vi "LoadEyeArray.vi"(0 "directory path of data and header file":path, 1 "Split files?":bool, 3 "Type of Read":T2(ring)=enum."Save IQSum", 5 "String":string="*_HeaderInfoRcv.txt", 7 "Only Buff 3?":bool, 12 "Only Real of Sum?":bool, 13 "Cut off":i32=50000) -> (4 "RcvBuff 3":cdb[][][](array[numeric]), 6 "output array":i32[][][](array[numeric]), 8 "Header Out":T1={"header info"={"Header"="", "Head length"=0}, "A/D info"={"# rf points per line"=0, "# lines per scan"=0, "sample rate MHz"=0, "# A/D bits"=0, "# bytes per A/D"=0, "TGC Flag"=0, "A/D Type"=""}, "Tranducer Info"={"bandwidth"=0.0, "center freq"=0.0, "start freq"=0.0, "ID"=0}, "Scan Info"={"delay"=0.0, "pivot distance"=0.0, "sector scan angle"=0.0, "operator"="", "Scan Mode"="", "location"=""}, "Time/Date Info"={"date"="", "time"=""}, "RF Info"={"RF file name"="", "RF file att"="", "RF cal file name"="", "RF cal file att"=""}, "Patient Info"={"ID"="", "extended ID"="", "age"=0, "sex"="", "previously\nscanned"="", "PSA"=0.0, "LOS"=1, "Ethnicty 2"=3, "Race"=3}, "Tissue Type"={"organ"=0, "disease type"=0, "disease location"=0, "IQ_pts"=0, "RcvBuffer"=0, "RcvFrame"=0, "IQBuff"=0, "IQFrame"=0, "IQPage"=0}, "Votage scaling"={"Digitizer (dB)"=0.0, "Gain (dB)"=0.0, "Atten (dB)"=0.0}, "Comment"="", "Misc Info"={"avg num"=0, "c speed"=0, "Div By or SF zones"=0, "XMIT CHS"=0, "RCV CHS"=0, "Xmit angle"=0.0}, "Therapy Parameters"={"Theraputic Freq (MHz)"=0.0, "Time on (s)"=0.0, "Therapy amplitude (mV)"=0.0, "Lines Before"=0, "Lines After"=0}, "Scan Settings"={"Energy (uJ or V)"=0, "Damp (Ohm) or Fc"=0, "HP Filt (KHz)"=0, "LP Filt (MHz)"=0, "Gain (db)"=0, "prf (kHz)"=0.0, "Distance between\nscan lines (um)"=0, "Distance between\nscan planes (um)"=0, "Scan line gap (um)"=0.0, "Scan plane gap (um)"=0.0}, "Compression Parameters"={"F1 (MHz)"=0.0, "F2 (MHz)"=0.0, "% taper"=0.0, "duration"=0.0}, "Patient Info Xtra"={"First Name"="", "Last Name"="", "Notes"=""}, "ROI Box"=[0, 0, 0, 0]} {"Compression Parameters"."% taper" min=50 max=1000 format="%.2f"; "Compression Parameters"."F2 (MHz)" format="%.3f"; "Compression Parameters"."F1 (MHz)" format="%.3f"; "Scan Settings"."prf (kHz)" format="%.2f"; "Therapy Parameters"."Therapy amplitude (mV)" min=50 max=1000 format="%.2f"; "Therapy Parameters"."Time on (s)" format="%.3f"; "Therapy Parameters"."Theraputic Freq (MHz)" format="%.3f"; "Patient Info"."Race" items=["Am Ind or Alaska", "Asian", "Hawaiian, Pac Isl", "Black or Afr Amer", "White", "more than one race", "unknown"]; "Patient Info"."Ethnicty 2" items=["Hispanic", "Non-Hispanic", "unknown"]; "Patient Info"."LOS" items=["1", "2", "3", "4", "5"]; "Patient Info"."PSA" format="%.1f"; "Scan Info"."delay" format="%.2f"; "Scan Info"."pivot distance" format="%.2f"; "Scan Info"."sector scan angle" format="%.2f"; "Tranducer Info"."bandwidth" format="%.2f"; "Tranducer Info"."center freq" format="%.2f"; "Tranducer Info"."start freq" format="%.2f"}, 10 "time diff (25 us time steps)":sgl[](graph), 15 "time stamp":sgl[](graph))   [LabVIEW 2022 SP3]
uses:
  ViewData/-ReadEye/Header.ctl
  <vilib>/Utility/file.llb/Read Delimited Spreadsheet (string).vi
  <vilib>/Utility/file.llb/Read Delimited Spreadsheet (DBL).vi
  <userlib>/_OpenG.lib/array/array.llb/Sort 2D Array (DBL)__ogtk.vi
panel:
  in  "#Sets":i32=1 min=1 max=100 step=1
  in  "Extra Char":string
  out "Raw data":dbl[][](graph)
  out "Current File":string
  in  "IQ source":enum32{"GPU", "Verasonics", "None"}(radio)
  out "Current File Ct":i32
  out "Header Size":i32[](array[numeric])
  out "Header clolumn names":string[](array[string])
  in  "Header as cluster":T3
  out "Header Values sorted":dbl[][](array[numeric])
  # "Naming must match up\nDo not change order in Matlab save !!!!!!!!!!!!!!!!!!!!!!!!!!!!!!"
  # "For LoopCT can add in _0n for the raw case"
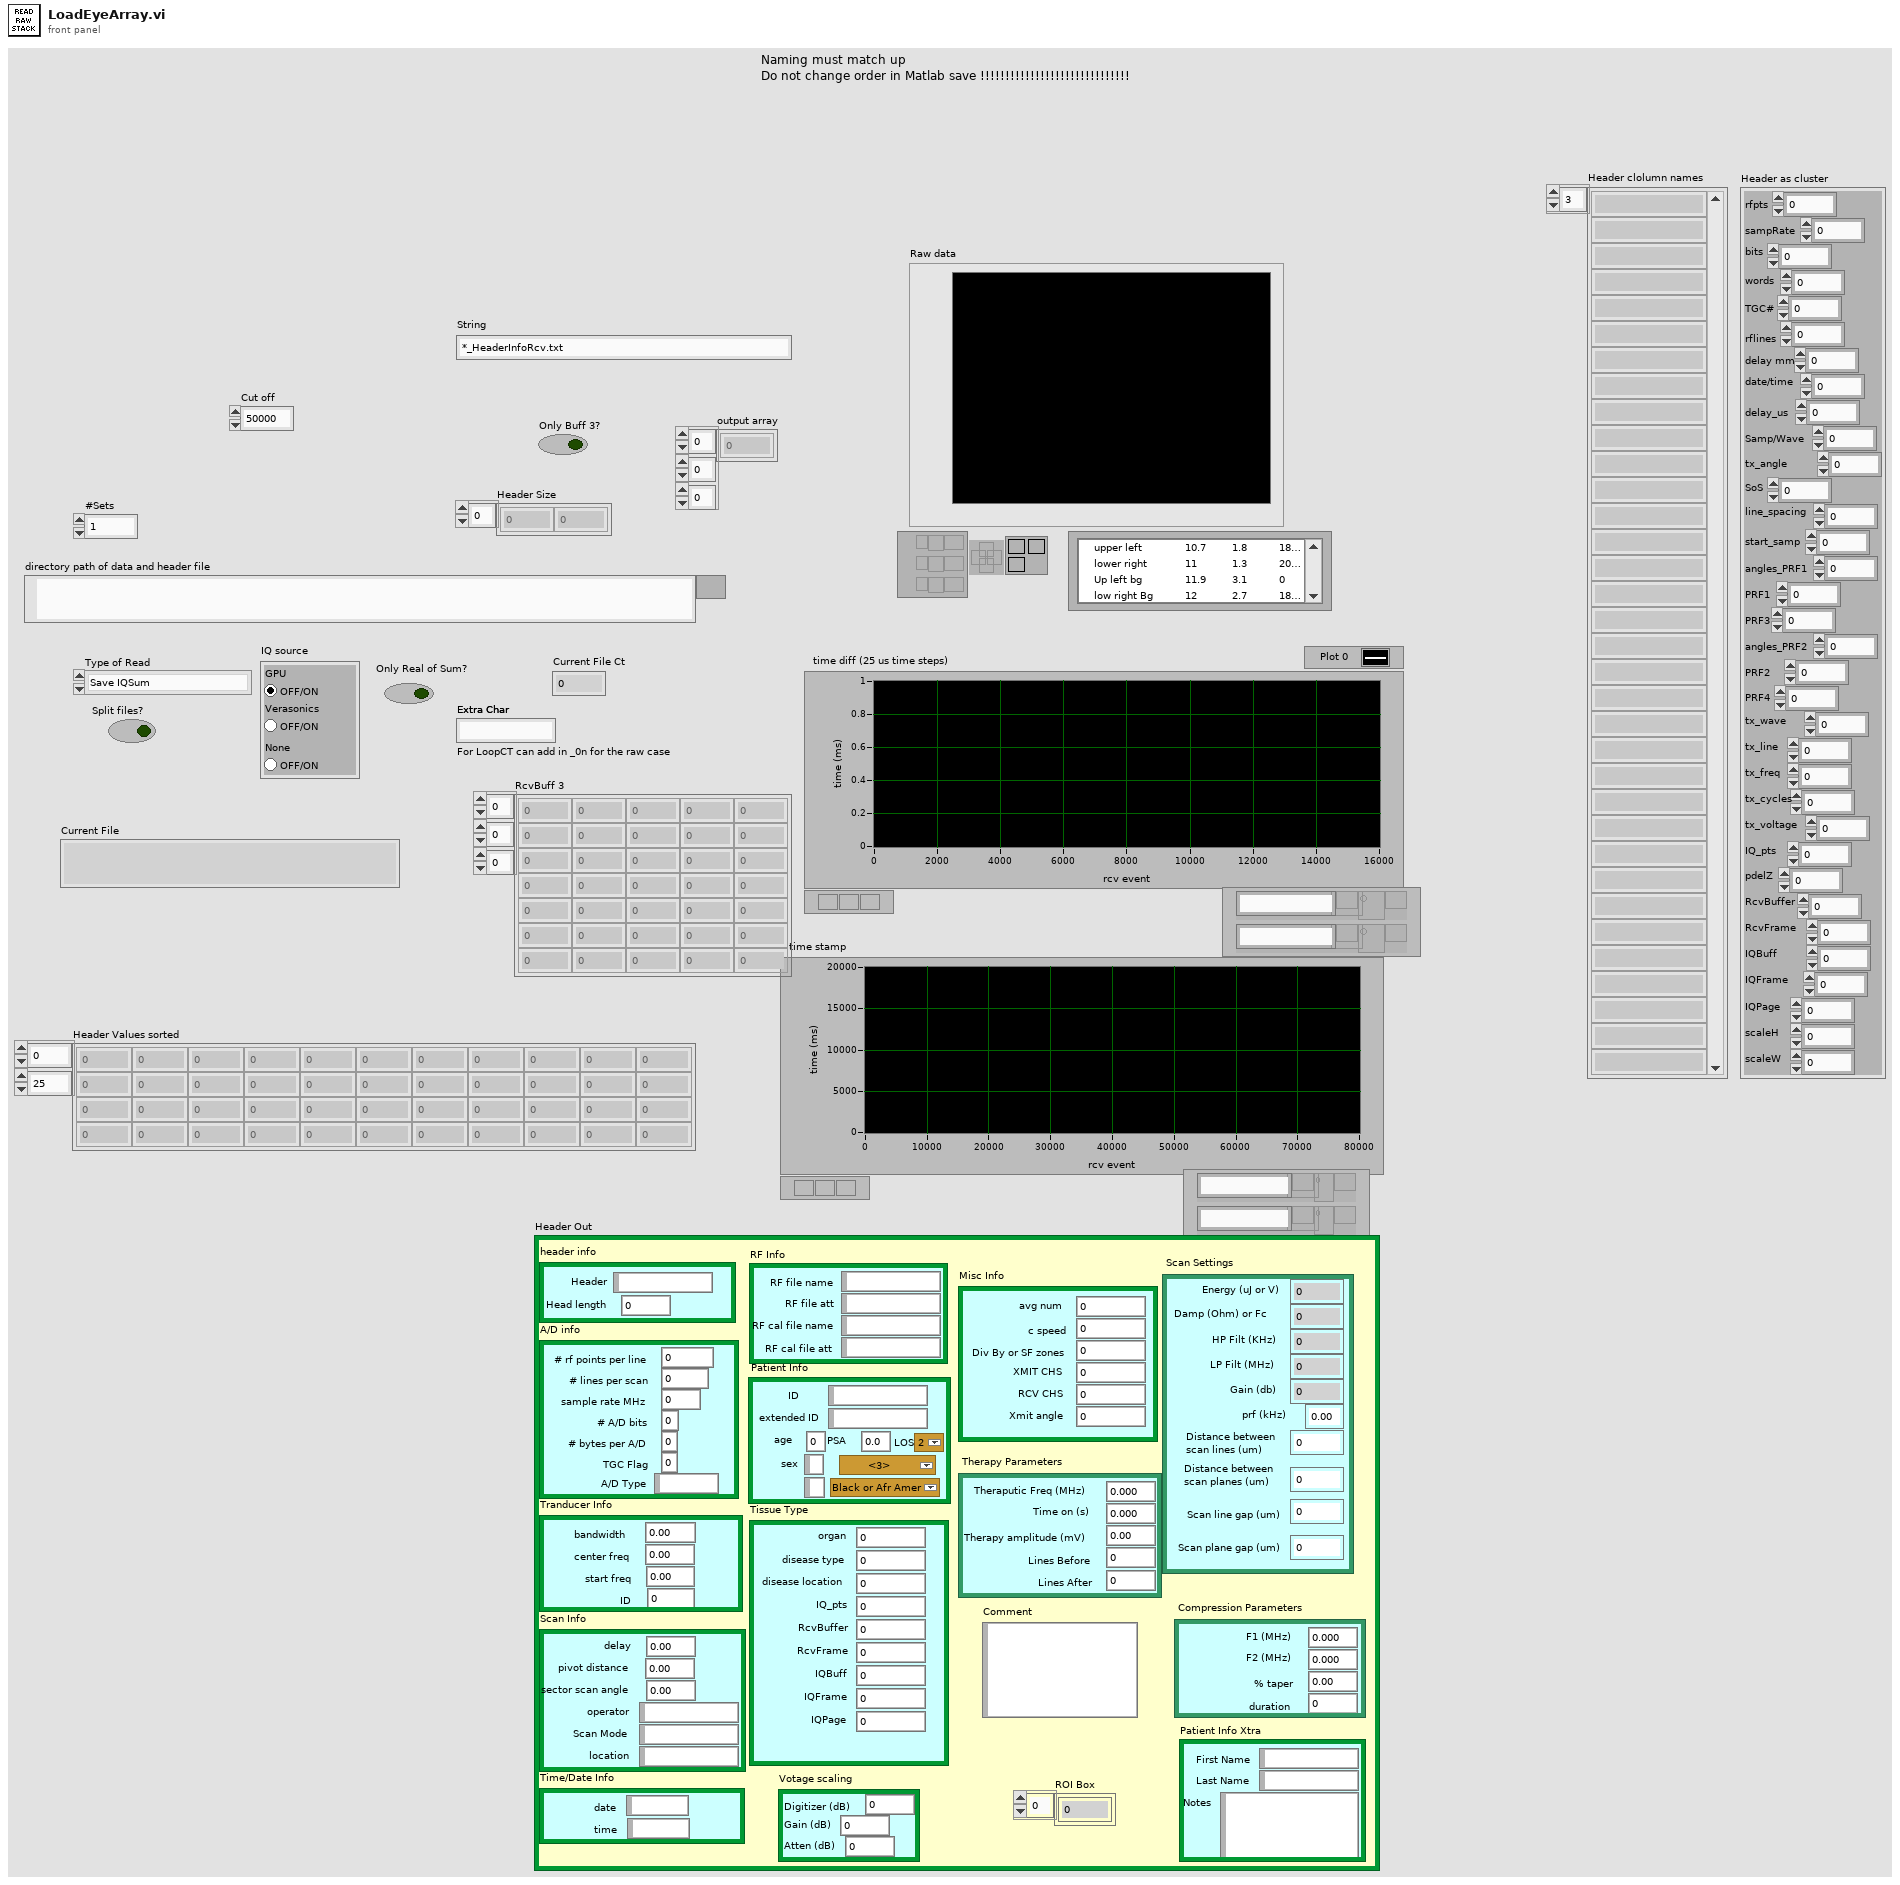
[diagram p1: front panel]
types:
  T1 = typedef "Header.ctl" = cluster{"header info":cluster{"Header":string, "Head length":i16}, "A/D info":cluster{"# rf points per line":u16, "# lines per scan":u16, "sample rate MHz":u16, "# A/D bits":i16, "# bytes per A/D":u16, "TGC Flag":u16, "A/D Type":string}, "Tranducer Info":cluster{"bandwidth":sgl, "center freq":sgl, "start freq":sgl, "ID":i32}, "Scan Info":cluster{"delay":sgl, "pivot distance":sgl, "sector scan angle":sgl, "operator":string, "Scan Mode":string, "location":string}, "Time/Date Info":cluster{"date":string, "time":string}, "RF Info":cluster{"RF file name":string, "RF file att":string, "RF cal file name":string, "RF cal file att":string}, "Patient Info":cluster{"ID":string, "extended ID":string, "age":u16, "sex":string, "previously\nscanned":string, "PSA":sgl, "LOS":u8, "Ethnicty 2":u8, "Race":u8}, "Tissue Type":cluster{"organ":i16, "disease type":i16, "disease location":i16, "IQ_pts":u16, "RcvBuffer":u8, "RcvFrame":u16, "IQBuff":u8, "IQFrame":u16, "IQPage":u8}, "Votage scaling":cluster{"Digitizer (dB)":sgl, "Gain (dB)":sgl, "Atten (dB)":sgl}, "Comment":string, "Misc Info":cluster{"avg num":u16, "c speed":i16, "Div By or SF zones":i16, "XMIT CHS":u8, "RCV CHS":u8, "Xmit angle":sgl}, "Therapy Parameters":cluster{"Theraputic Freq (MHz)":sgl, "Time on (s)":sgl, "Therapy amplitude (mV)":sgl, "Lines Before":u16, "Lines After":u16}, "Scan Settings":cluster{"Energy (uJ or V)":u8, "Damp (Ohm) or Fc":u8, "HP Filt (KHz)":u8, "LP Filt (MHz)":u8, "Gain (db)":u8, "prf (kHz)":sgl, "Distance between\nscan lines (um)":u16, "Distance between\nscan planes (um)":u16, "Scan line gap (um)":sgl, "Scan plane gap (um)":sgl}, "Compression Parameters":cluster{"F1 (MHz)":sgl, "F2 (MHz)":sgl, "% taper":sgl, "duration":sgl}, "Patient Info Xtra":cluster{"First Name":string, "Last Name":string, "Notes":string}, "ROI Box":u16[]}
  T2 = enum16{"None", "Raw RF + time stamp", "Save IQAll", "Save IQSum", "Save IQSumReal", "Save Img", "Time Stamps", "unused"}
  T3 = cluster{"rfpts":dbl, "sampRate":dbl, "bits":dbl, "words":dbl, "TGC#":dbl, "rflines":dbl, "delay mm":dbl, "date/time":dbl, "delay_us":dbl, "Samp/Wave":dbl, "tx_angle":dbl, "SoS":dbl, "line_spacing":dbl, "start_samp":dbl, "angles_PRF1":dbl, "PRF1":dbl, "PRF3":dbl, "angles_PRF2":dbl, "PRF2":dbl, "PRF4":dbl, "tx_wave":dbl, "tx_line":dbl, "tx_freq":dbl, "tx_cycles":dbl, "tx_voltage":dbl, "IQ_pts":dbl, "pdelZ":dbl, "RcvBuffer":dbl, "RcvFrame":dbl, "IQBuff":dbl, "IQFrame":dbl, "IQPage":dbl, "scaleH":dbl, "scaleW":dbl}
  T4 = enum16{"big-endian, network order", "native, host order", "little-endian"}
  T5 = cluster{"Sorted Array out[0]":dbl, "Sorted Array out[1]":dbl, "Sorted Array out[2]":dbl, "Sorted Array out[3]":dbl, "Sorted Array out[4]":dbl, "Sorted Array out[5]":dbl, "Sorted Array out[6]":dbl, "Sorted Array out[7]":dbl, "Sorted Array out[8]":dbl, "Sorted Array out[9]":dbl, "Sorted Array out[10]":dbl, "Sorted Array out[11]":dbl, "Sorted Array out[12]":dbl, "Sorted Array out[13]":dbl, "Sorted Array out[14]":dbl, "Sorted Array out[15]":dbl, "Sorted Array out[16]":dbl, "Sorted Array out[17]":dbl, "Sorted Array out[18]":dbl, "Sorted Array out[19]":dbl, "Sorted Array out[20]":dbl, "Sorted Array out[21]":dbl, "Sorted Array out[22]":dbl, "Sorted Array out[23]":dbl, "Sorted Array out[24]":dbl, "Sorted Array out[25]":dbl, "Sorted Array out[26]":dbl, "Sorted Array out[27]":dbl, "Sorted Array out[28]":dbl, "Sorted Array out[29]":dbl, "Sorted Array out[30]":dbl, "Sorted Array out[31]":dbl, "Sorted Array out[32]":dbl, "Sorted Array out[33]":dbl, "Sorted Array out[34]":dbl}
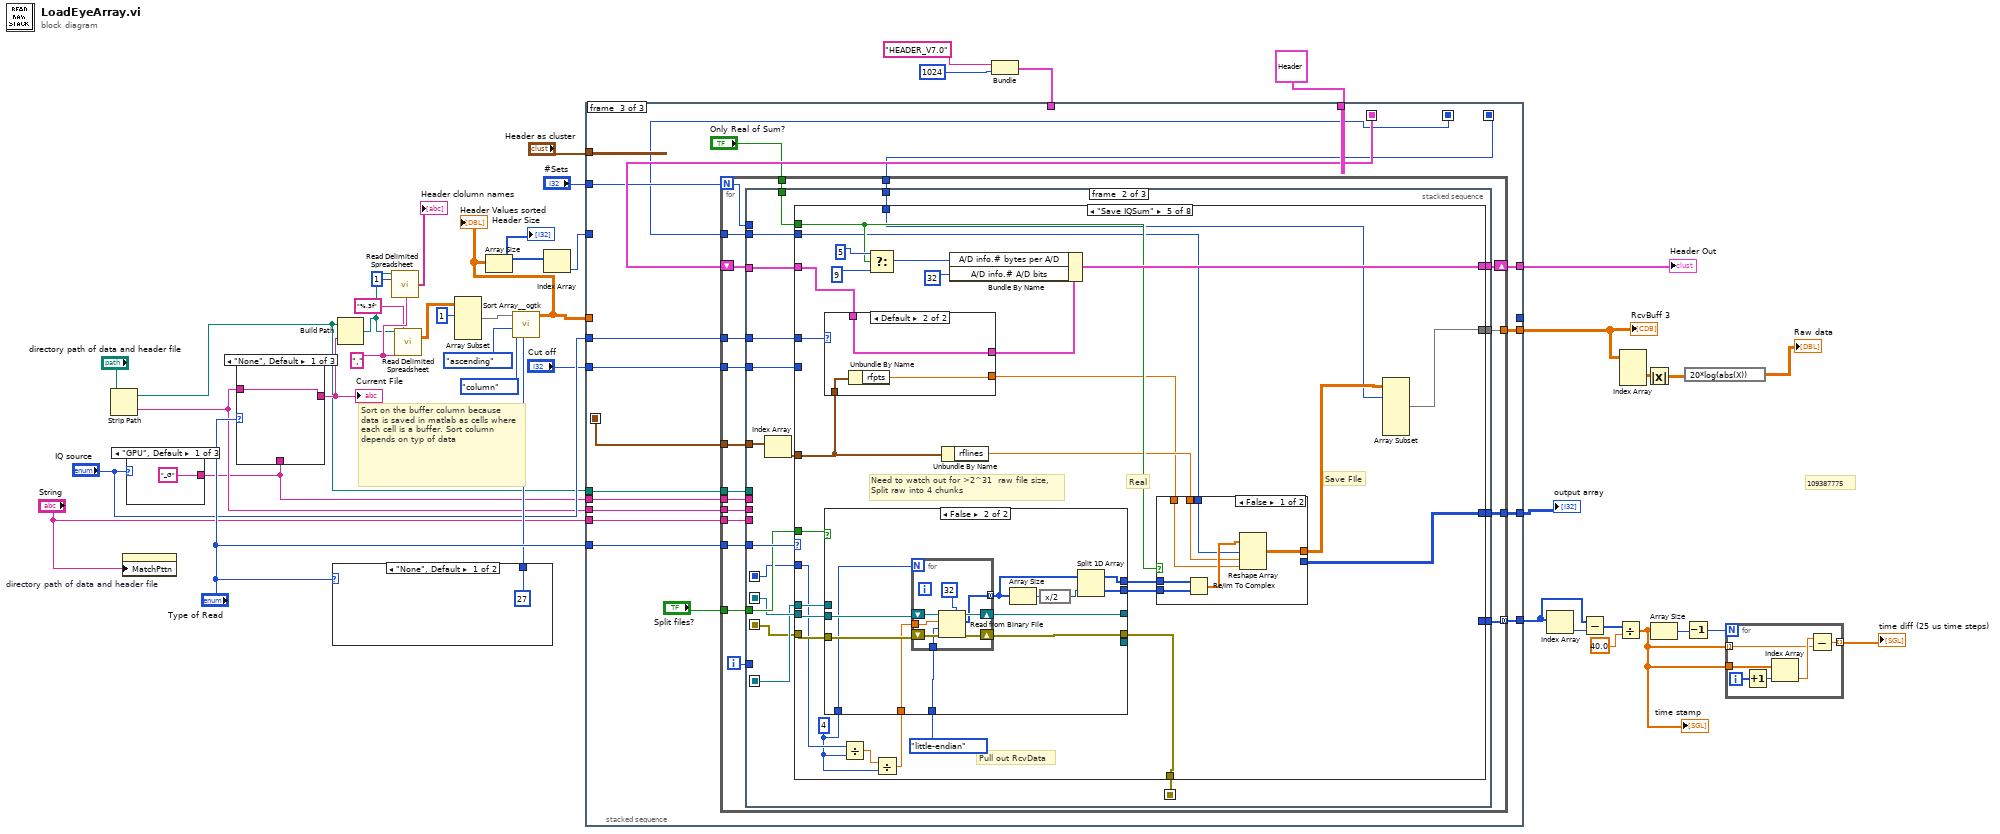
[diagram p0: block diagram]
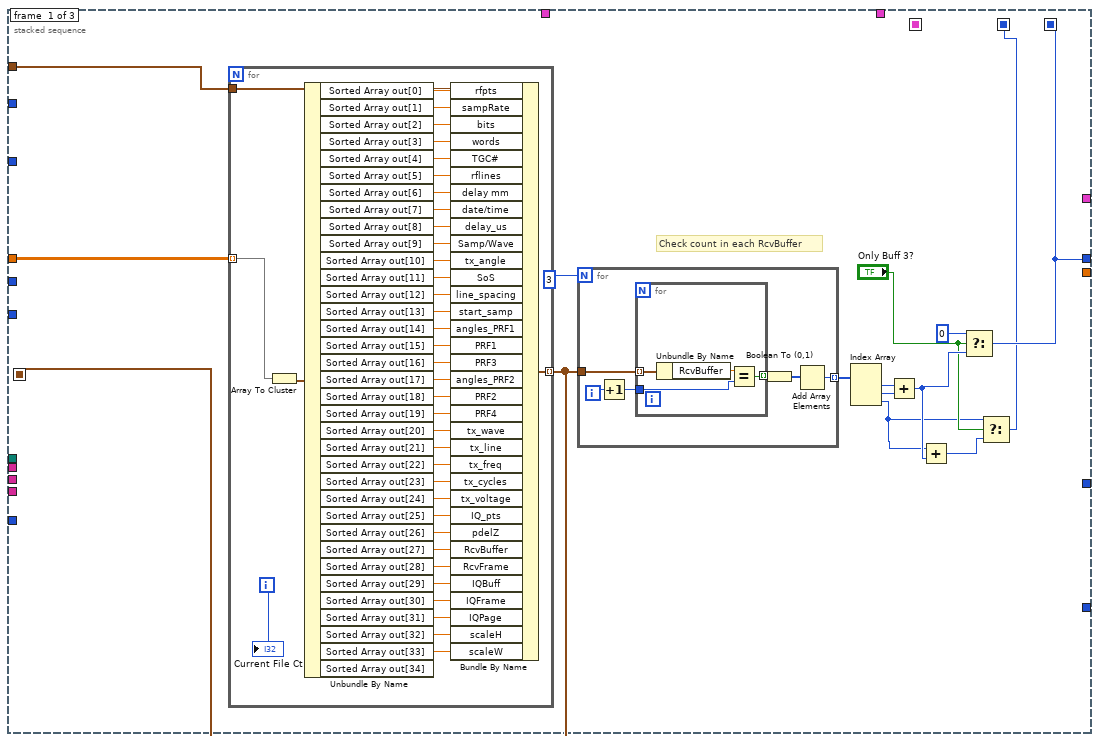
[diagram p2: hidden frame]
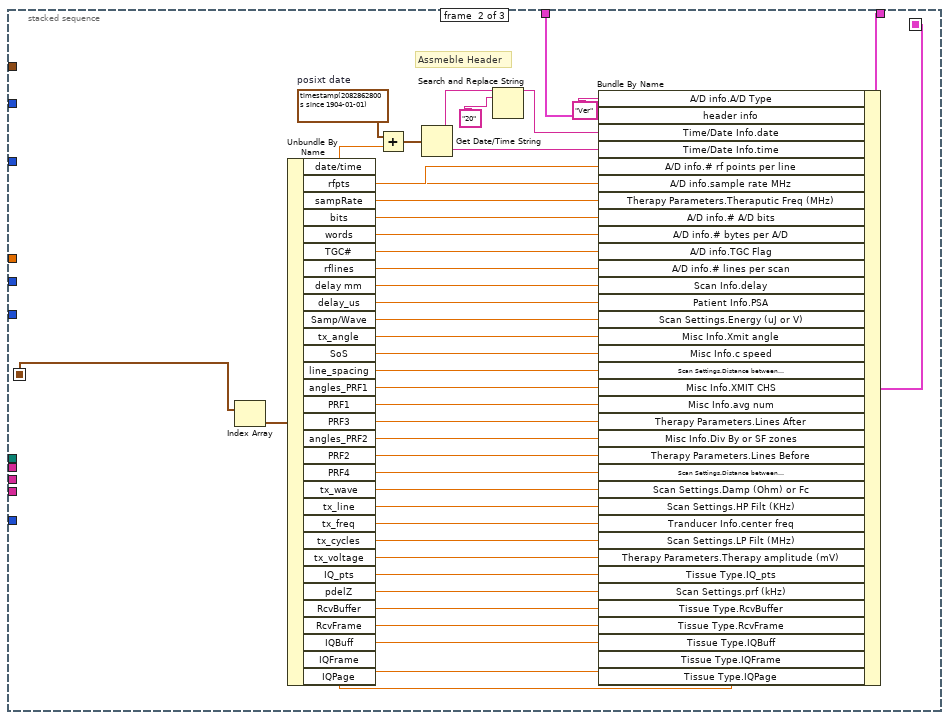
[diagram p3: hidden frame]
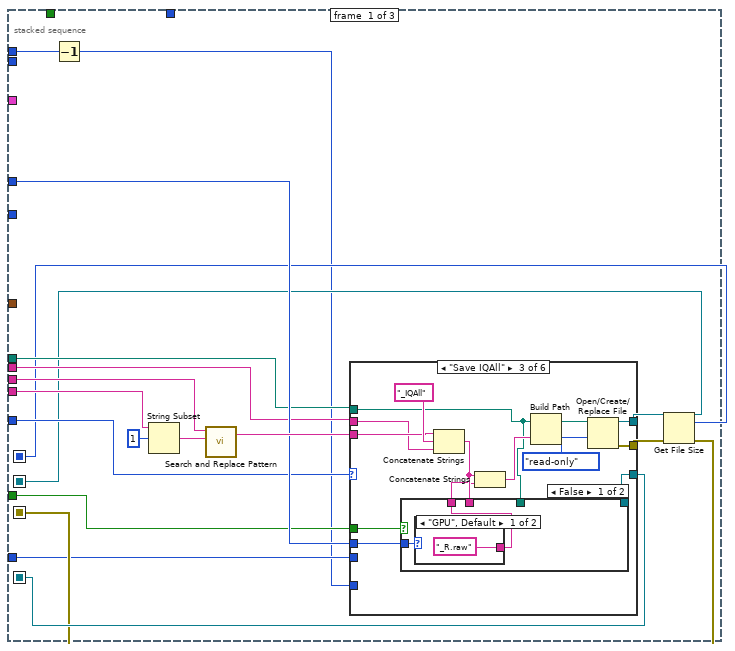
[diagram p4: hidden frame]
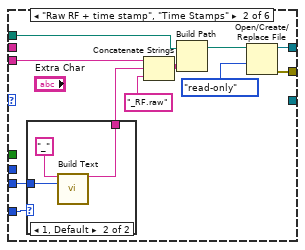
[diagram p6: hidden frame]
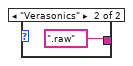
[diagram p8: hidden frame]
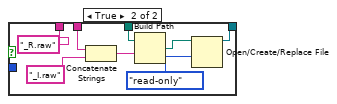
[diagram p9: hidden frame]
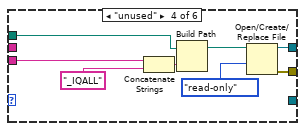
[diagram p10: hidden frame]
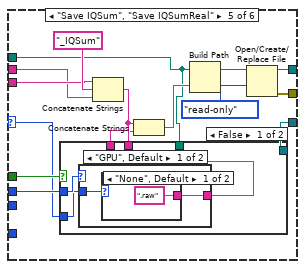
[diagram p11: hidden frame]
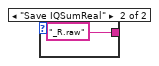
[diagram p12: hidden frame]
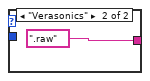
[diagram p13: hidden frame]
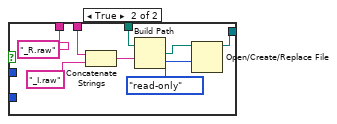
[diagram p14: hidden frame]
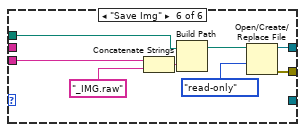
[diagram p15: hidden frame]
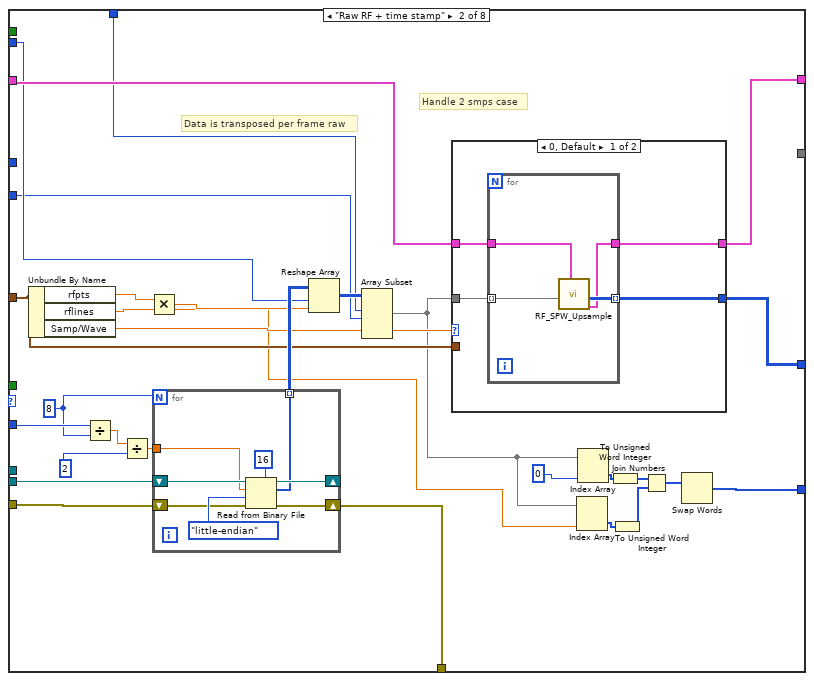
[diagram p17: hidden frame]
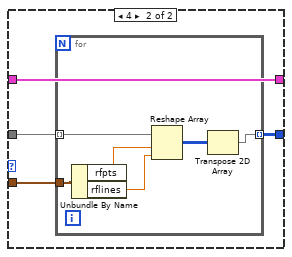
[diagram p18: hidden frame]
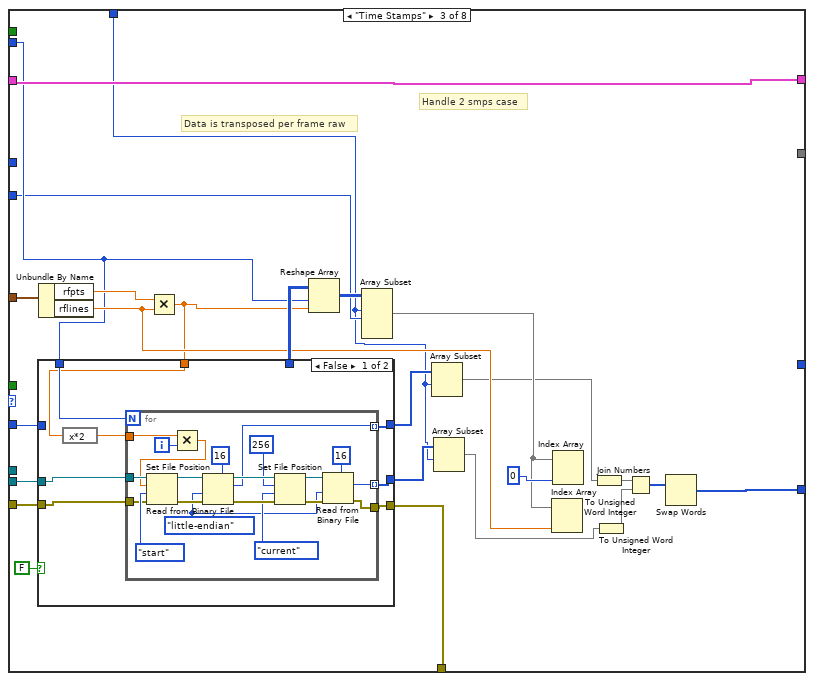
[diagram p19: hidden frame]
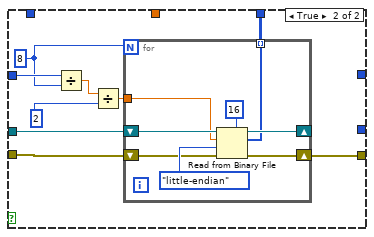
[diagram p20: hidden frame]
diagram:
  w34 = "," ("delimiter (\\t)")
  # "109387775"
  # "Sort on the buffer column because data is saved in matlab as cells where each cell is a buffer. Sort column depends on typ of data"
  n1 = Strip Path(path="directory path of data and header file") -> (stripped path=w11:path, name=w13:string)
  n2 = property on="directory path of data and header file" class="Path"("MatchPttn"="String") -> ()  [unwired: 2 in, 2 out]
  n3 = case shown="\"GPU\", Default" "IQ source" {
    tunnel: ["_G" ("replace string (\"\")") "_V" ("replace string (\"\")") _] -> w12
    frame "GPU", Default {
    }
    frame "Verasonics" {
    }
    frame "None" {
    }
  }
  n4 = case shown="\"None\", Default" "Type of Read" {
    tunnel: w13 -> [w46 w51 w57]
    tunnel: [w46 w50 w56] -> w31
    tunnel: w12 -> [_ w47 w53]
    frame "None", Default {
    }
    frame "Save IQSum".."Save Img" {
      n5 = Concatenate Strings("IQSum" ("replace string (\"\")"), w47) -> (w48:string)
      n6 = Search and Replace String(input string=w51, search string="Rcv", replace string=w48) -> (result string=w50:string)  [unwired: 5 in, 3 out]
    }
    frame "Save IQAll" {
      n7 = Concatenate Strings("IQAll" ("replace string (\"\")"), w53) -> (w54:string)
      n8 = Search and Replace String(input string=w57, search string="Rcv", replace string=w54) -> (result string=w56:string)  [unwired: 5 in, 3 out]
    }
  }
  "Current File" <- w31
  n9 = case shown="\"None\", Default" "Type of Read" {
    tunnel: [u32 27 ("Column/Row to Sort By") u32 29 ("Column/Row to Sort By")] -> w26
    frame "None", Default {
    }
    frame "Save IQSum".."Save Img" {
    }
  }
  n10 = Build Path(base path=w11, name or relative path=w31) -> (appended path=w23:path)
  n11 = call-poly <vilib>:"Read Delimited Spreadsheet.vi"("file path (dialog if empty)"=w23, "number of rows (all:-1)"=1, "delimiter (\\t)"=w34) -> ("first row"=→"Header clolumn names":string[])  [unwired: 7 in, 5 out]
  n12 = call-poly <vilib>:"Read Delimited Spreadsheet.vi"("file path (dialog if empty)"=w23, "format (%.3f)"="%.3f", "delimiter (\\t)"=w34) -> ("all rows"=w37:dbl[][])  [unwired: 7 in, 5 out]
  n13 = Array Subset(array=w37, index (row)=1 ("index")) -> (w28:dbl[][])  [unwired: 3 in]
  n14 = call-poly <userlib>:"Sort Array__ogtk.vi"("Column/Row to Sort By"=w26, "Sort By in"=enum16{"row", "column"}."column", "Order"=enum16{"ascending", "descending"}."ascending", "Array in"=w28) -> ("Sorted Array out"=w27:dbl[][])  [unwired: 4 in, 3 out]
  "Header Values sorted" <- w27
  n15 = Array Size(array=w27) -> (size(s)=w22:i32[])
  "Header Size" <- w22
  n16 = Index Array(array=w22) -> (element=w9:i32)  [unwired: 1 in]
  n17 = Bundle("HEADER_V7.0", 1024) -> (w40:cluster{string, i32})  [unwired: 1 in]
  n18 = stacked-sequence {
    seq-local: [_ w135 _] -> [_ _ w184]
    seq-local: [w71 _ _] -> [_ w125 w177]
    seq-local: [w65 _ _] -> [_ _ w176]
    seq-local: [w61 _ _] -> [_ _ w167]
    tunnel: T1 {"header info"={"Header"="", "Head length"=0}, "A/D info"={"# rf points per line"=0, "# lines per scan"=0, "sample rate MHz"=0, "# A/D bits"=0, "# bytes per A/D"=0, "TGC Flag"=0, "A/D Type"=""}, "Tranducer Info"={"bandwidth"=0.0, "center freq"=0.0, "start freq"=0.0, "ID"=0}, "Scan Info"={"delay"=0.0, "pivot distance"=0.0, "sector scan angle"=0.0, "operator"="", "Scan Mode"="", "location"=""}, "Time/Date Info"={"date"="", "time"=""}, "RF Info"={"RF file name"="", "RF file att"="", "RF cal file name"="", "RF cal file att"=""}, "Patient Info"={"ID"="", "extended ID"="", "age"=0, "sex"="", "previously\nscanned"="", "PSA"=0.0, "LOS"=1, "Ethnicty 2"=3, "Race"=3}, "Tissue Type"={"organ"=0, "disease type"=0, "disease location"=0, "IQ_pts"=0, "RcvBuffer"=0, "RcvFrame"=0, "IQBuff"=0, "IQFrame"=0, "IQPage"=0}, "Votage scaling"={"Digitizer (dB)"=0.0, "Gain (dB)"=0.0, "Atten (dB)"=0.0}, "Comment"="", "Misc Info"={"avg num"=0, "c speed"=0, "Div By or SF zones"=0, "XMIT CHS"=0, "RCV CHS"=0, "Xmit angle"=0.0}, "Therapy Parameters"={"Theraputic Freq (MHz)"=0.0, "Time on (s)"=0.0, "Therapy amplitude (mV)"=0.0, "Lines Before"=0, "Lines After"=0}, "Scan Settings"={"Energy (uJ or V)"=0, "Damp (Ohm) or Fc"=0, "HP Filt (KHz)"=0, "LP Filt (MHz)"=0, "Gain (db)"=0, "prf (kHz)"=0.0, "Distance between\nscan lines (um)"=0, "Distance between\nscan planes (um)"=0, "Scan line gap (um)"=0.0, "Scan plane gap (um)"=0.0}, "Compression Parameters"={"F1 (MHz)"=0.0, "F2 (MHz)"=0.0, "% taper"=0.0, "duration"=0.0}, "Patient Info Xtra"={"First Name"="", "Last Name"="", "Notes"=""}, "ROI Box"=[0, 0, 0, 0]} ("Header In") -> [_ w166 _]
    tunnel: w40 -> [_ w140 _]
    tunnel: "Type of Read" -> [_ _ w183]
    tunnel: w27 -> [w74 _ _]
    tunnel: "Header as cluster" -> [w73 _ _]
    tunnel: "IQ source" -> [_ _ w182]
    tunnel: [_ _ w180] -> w38
    tunnel: w9 -> [_ _ _]
    tunnel: [_ _ w179] -> w20
    tunnel: [_ _ w178] -> w19
    tunnel: [w65 _ _] -> _
    tunnel: "Cut off" -> [_ _ w175]
    tunnel: "String" -> [_ _ w174]
    tunnel: w13 -> [_ _ w173]
    tunnel: w12 -> [_ _ w172]
    tunnel: w11 -> [_ _ w171]
    tunnel: "#Sets" -> [_ _ w170]
    tunnel: [_ _ w168] -> w3
    frame #0 {
      # "Check count in each RcvBuffer"
      n19 = for {
        tunnel: w74 -> [w91] mode=indexing
        tunnel: w73 -> [w86]
        tunnel: [w85] -> w71 mode=indexing
        i -> [w87]
        n20 = Array To Cluster(array=w91) -> (cluster=w90:T5)
        n21 = Unbundle By Name(w90) -> ("Sorted Array out[0]"=w123:dbl, "Sorted Array out[1]"=w122:dbl, "Sorted Array out[2]"=w121:dbl, "Sorted Array out[3]"=w120:dbl, "Sorted Array out[4]"=w119:dbl, "Sorted Array out[5]"=w118:dbl, "Sorted Array out[6]"=w117:dbl, "Sorted Array out[7]"=w116:dbl, "Sorted Array out[8]"=w115:dbl, "Sorted Array out[9]"=w114:dbl, "Sorted Array out[10]"=w113:dbl, "Sorted Array out[11]"=w112:dbl, "Sorted Array out[12]"=w111:dbl, "Sorted Array out[13]"=w110:dbl, "Sorted Array out[14]"=w109:dbl, "Sorted Array out[15]"=w108:dbl, "Sorted Array out[16]"=w107:dbl, "Sorted Array out[17]"=w106:dbl, "Sorted Array out[18]"=w105:dbl, "Sorted Array out[19]"=w104:dbl, "Sorted Array out[20]"=w103:dbl, "Sorted Array out[21]"=w102:dbl, "Sorted Array out[22]"=w101:dbl, "Sorted Array out[23]"=w100:dbl, "Sorted Array out[24]"=w99:dbl, "Sorted Array out[25]"=w98:dbl, "Sorted Array out[26]"=w97:dbl, "Sorted Array out[27]"=w96:dbl, "Sorted Array out[28]"=w95:dbl, "Sorted Array out[29]"=w92:dbl, "Sorted Array out[30]"=w93:dbl, "Sorted Array out[31]"=w94:dbl, "Sorted Array out[32]"=w89:dbl, "Sorted Array out[33]"=w88:dbl)  [unwired: 1 out]
        n22 = Bundle By Name(cluster=w86, "rfpts"=w123, "sampRate"=w122, "bits"=w121, "words"=w120, "TGC#"=w119, "rflines"=w118, "delay mm"=w117, "date/time"=w116, "delay_us"=w115, "Samp/Wave"=w114, "tx_angle"=w113, "SoS"=w112, "line_spacing"=w111, "start_samp"=w110, "angles_PRF1"=w109, "PRF1"=w108, "PRF3"=w107, "angles_PRF2"=w106, "PRF2"=w105, "PRF4"=w104, "tx_wave"=w103, "tx_line"=w102, "tx_freq"=w101, "tx_cycles"=w100, "tx_voltage"=w99, "IQ_pts"=w98, "pdelZ"=w97, "RcvBuffer"=w96, "RcvFrame"=w95, "IQBuff"=w92, "IQFrame"=w93, "IQPage"=w94, "scaleH"=w89, "scaleW"=w88) -> (w85:T3)
        "Current File Ct" <- w87
      }
      n23 = for {
        N: 3 -> [_]
        tunnel: w71 -> [w80]
        tunnel: [w75] -> w70 mode=indexing
        i -> [w79]
        n24 = Increment(x=w79) -> (x+1=w78:i32)
        n25 = for {
          tunnel: w80 -> [w84] mode=indexing
          tunnel: w78 -> [w83]
          tunnel: [w81] -> w77 mode=indexing
          n26 = Unbundle By Name(w84) -> ("RcvBuffer"=w82:dbl)
          n27 = Equal?(x=w82, y=w83) -> (x = y?=w81:bool)
        }
        n28 = Boolean To (0,1)(Boolean=w77) -> (0, 1=w76:i16[])
        n29 = Add Array Elements(numeric array=w76) -> (sum=w75:i16)
      }
      n30 = Index Array(array=w70) -> (element #1=w69:i16, element #2=w68:i16, element #3=w63:i16)  [unwired: 3 in]
      n31 = Add(x=w69, y=w68) -> (x+y=w67:i16)
      n32 = Add(x=w63, y=w67) -> (x+y=w62:i16)
      n33 = Select(t=i16 0, s="Only Buff 3?", f=w67) -> (s? t:f=w65:i16)
      n34 = Select(t=w63, s="Only Buff 3?", f=w62) -> (s? t:f=w61:i16)
    }
    frame #1 {
      w151 = timestamp(2082862800 s since 1904-01-01)  # posixt date
      # "Assmeble Header"
      n35 = Index Array(array=w125) -> (element=w124:T3)  [unwired: 1 in]
      n36 = Unbundle By Name(w124) -> ("date/time"=w152:dbl, "rfpts"=w128:dbl, "sampRate"=w127:dbl, "bits"=w147:dbl, "words"=w165:dbl, "TGC#"=w164:dbl, "rflines"=w163:dbl, "delay mm"=w162:dbl, "delay_us"=w161:dbl, "Samp/Wave"=w160:dbl, "tx_angle"=w141:dbl, "SoS"=w155:dbl, "line_spacing"=w142:dbl, "angles_PRF1"=w159:dbl, "PRF1"=w146:dbl, "PRF3"=w158:dbl, "angles_PRF2"=w156:dbl, "PRF2"=w157:dbl, "PRF4"=w145:dbl, "tx_wave"=w144:dbl, "tx_line"=w143:dbl, "tx_freq"=w139:dbl, "tx_cycles"=w138:dbl, "tx_voltage"=w137:dbl, "IQ_pts"=w134:dbl, "pdelZ"=w133:dbl, "RcvBuffer"=w126:dbl, "RcvFrame"=w132:dbl, "IQBuff"=w131:dbl, "IQFrame"=w130:dbl, "IQPage"=w129:dbl)
      n37 = Add(x=w151, y=w152) -> (x+y=w154:timestamp)
      n38 = Get Date/Time String(seconds (now)=w154) -> (date string=w150:string, time string=w153:string)  [unwired: 2 in]
      n39 = Search and Replace String(input string=w150, search string="20") -> (result string=w148:string)  [unwired: 2 in, 7 out]
      n40 = Bundle By Name(cluster=w166, "A/D info.A/D Type"="Ver", "header info"=w140, "Time/Date Info.date"=w148, "Time/Date Info.time"=w153, "A/D info.# rf points per line"=w128, "A/D info.sample rate MHz"=w127, "Therapy Parameters.Theraputic Freq (MHz)"=w127, "A/D info.# A/D bits"=w147, "A/D info.# bytes per A/D"=w165, "A/D info.TGC Flag"=w164, "A/D info.# lines per scan"=w163, "Scan Info.delay"=w162, "Patient Info.PSA"=w161, "Scan Settings.Energy (uJ or V)"=w160, "Misc Info.Xmit angle"=w141, "Misc Info.c speed"=w155, "Scan Settings.Distance between\nscan lines (um)"=w142, "Misc Info.XMIT CHS"=w159, "Misc Info.avg num"=w146, "Therapy Parameters.Lines After"=w158, "Misc Info.Div By or SF zones"=w156, "Therapy Parameters.Lines Before"=w157, "Scan Settings.Distance between\nscan planes (um)"=w145, "Scan Settings.Damp (Ohm) or Fc"=w144, "Scan Settings.HP Filt (KHz)"=w143, "Tranducer Info.center freq"=w139, "Scan Settings.LP Filt (MHz)"=w138, "Therapy Parameters.Therapy amplitude (mV)"=w137, "Tissue Type.IQ_pts"=w134, "Scan Settings.prf (kHz)"=w133, "Tissue Type.RcvBuffer"=w126, "Tissue Type.RcvFrame"=w132, "Tissue Type.IQBuff"=w131, "Tissue Type.IQFrame"=w130, "Tissue Type.IQPage"=w129) -> (w135:T1)
    }
    frame #2 {
      n41 = for {
        N: w170 -> [w185]
        tunnel: w183 -> [w202]
        tunnel: "Split files?" -> [w201]
        tunnel: w182 -> [w200]
        tunnel: "Only Real of Sum?" -> [w199]
        tunnel: w167 -> [w197]
        tunnel: [w196] -> w179
        tunnel: [w195] -> w178
        tunnel: w177 -> [w194]
        tunnel: w176 -> [w193]
        tunnel: w175 -> [w192]
        shift-right: [w198] -> w180
        shift-left: w184 -> [w203]
        tunnel: w174 -> [w191]
        tunnel: w173 -> [w190]
        tunnel: w172 -> [w189]
        tunnel: w171 -> [w188]
        tunnel: [w187] -> w168 mode=concatenating
        i -> [w186]
        n42 = stacked-sequence {
          seq-local: [w209 _ _] -> [_ w315 w686]
          seq-local: [w210 _ _] -> [_ w314 w687]
          seq-local: [w208 _ _] -> [_ w313 w685]
          seq-local: [w207 _ _] -> [_ w312 _]
          seq-local: [_ w311 _] -> [_ _ _]
          tunnel: w203 -> [_ w328 _]
          tunnel: w202 -> [w214 w327 w689]
          tunnel: w201 -> [w212 w326 w688]
          tunnel: w200 -> [w217 w325 _]
          tunnel: w199 -> [_ w324 _]
          tunnel: [_ w323 _] -> w198
          tunnel: w197 -> [_ w322 _]
          tunnel: [_ w321 _] -> w196
          tunnel: [_ w320 _] -> w195
          tunnel: w194 -> [_ w319 _]
          tunnel: w193 -> [_ w317 _]
          tunnel: w192 -> [_ w316 _]
          tunnel: w191 -> [w216 _ _]
          tunnel: w190 -> [w215 _ _]
          tunnel: w189 -> [w213 _ _]
          tunnel: w188 -> [w211 _ _]
          tunnel: [_ w310 _] -> w187
          tunnel: w186 -> [w206 _ _]
          tunnel: w185 -> [w205 _ _]
          frame #0 {
            n43 = Decrement(x=w205) -> (x-1=w204:i32)
            n44 = String Subset(string=w216, offset (0)=1) -> (substring=w222:string)  [unwired: 1 in]
            n45 = call <vilib>:"Search and Replace Pattern.vi"("string"=w215, "regular expression (\"\")"=w222) -> ("result string"=w220:string)  [unwired: 3 in, 1 out]
            n46 = case shown="\"Save IQAll\"" w214 {
              selector: w214 -> [_ _ _ _ w271 _]
              tunnel: w220 -> [_ w232 w249 w268 w284 w307]
              tunnel: [_ w230 w247 w266 w282 w305] -> w219
              tunnel: [_ w229 w246 w265 w281 w304] -> w218
              tunnel: w211 -> [_ w227 w241 w263 w276 w302]
              tunnel: w213 -> [_ _ w244 _ w279 _]
              tunnel: [_ _ w240 _ w275 _] -> w210
              tunnel: w212 -> [_ _ w239 _ w274 _]
              tunnel: w217 -> [_ _ w237 _ w272 _]
              tunnel: w206 -> [_ w226 _ _ _ _]
              tunnel: w204 -> [_ w224 _ _ _ _]
              frame "None", Default {
              }
              frame "Raw RF + time stamp", "Time Stamps" {
                n47 = case shown="1, Default" w224 {
                  tunnel: w226 -> [_ w236]
                  tunnel: [_ w235] -> w223
                  frame 0 {
                  }
                  frame 1, Default {
                    n48 = call "Build Text"("Beginning Text"="_", "s"=w236) -> ("Result"=w235:string)  [unwired: 12 in, 1 out]
                  }
                }
                n49 = Concatenate Strings(w232, w223, "_RF.raw") -> (w233:string)
                n50 = Build Path(base path=w227, name or relative path=w233) -> (appended path=w231:path)
                n51 = Open/Create/Replace File(file path (use dialog)=w231, access (0:read/write)=enum16{"read/write", "read-only", "write-only"}."read-only") -> (refnum out=w230:refnum<file>, error out=w229:errorcluster)  [unwired: 4 in, 1 out]
              }
              frame "Save IQAll" {
                n52 = Concatenate Strings(w249, "_IQAll", w244) -> (w243:string)
                n53 = case shown="False" w239 {
                  tunnel: w243 -> [_ w262]
                  tunnel: w241 -> [_ w258]
                  tunnel: [_ w256] -> w240
                  tunnel: [w251 "_R.raw"] -> w238
                  tunnel: w237 -> [w252 _]
                  frame False {
                    n54 = case shown="\"GPU\", Default" w252 {
                      tunnel: ["_R.raw" ".raw"] -> w251
                      frame "GPU", Default {
                      }
                      frame "Verasonics" {
                      }
                    }
                  }
                  frame True {
                    n55 = Concatenate Strings(w262, "_I.raw") -> (w259:string)
                    n56 = Build Path(base path=w258, name or relative path=w259) -> (appended path=w257:path)
                    n57 = Open/Create/Replace File(file path (use dialog)=w257, access (0:read/write)=enum16{"read/write", "read-only", "write-only"}."read-only") -> (refnum out=w256:refnum<file>)  [unwired: 4 in, 2 out]
                  }
                }
                n58 = Concatenate Strings(w243, w238) -> (w242:string)
                n59 = Build Path(base path=w241, name or relative path=w242) -> (appended path=w248:path)
                n60 = Open/Create/Replace File(file path (use dialog)=w248, access (0:read/write)=enum16{"read/write", "read-only", "write-only"}."read-only") -> (refnum out=w247:refnum<file>, error out=w246:errorcluster)  [unwired: 4 in, 1 out]
              }
              frame "unused" {
                n61 = Concatenate Strings(w268, "_IQALL") -> (w270:string)
                n62 = Build Path(base path=w263, name or relative path=w270) -> (appended path=w267:path)
                n63 = Open/Create/Replace File(file path (use dialog)=w267, access (0:read/write)=enum16{"read/write", "read-only", "write-only"}."read-only") -> (refnum out=w266:refnum<file>, error out=w265:errorcluster)  [unwired: 4 in, 1 out]
              }
              frame "Save IQSum", "Save IQSumReal" {
                n64 = Concatenate Strings(w284, "_IQSum", w279) -> (w278:string)
                n65 = case shown="False" w274 {
                  tunnel: w278 -> [_ w301]
                  tunnel: w276 -> [_ w297]
                  tunnel: [_ w295] -> w275
                  tunnel: [w287 "_R.raw"] -> w273
                  tunnel: w272 -> [w288 _]
                  tunnel: w271 -> [w286 _]
                  frame False {
                    n66 = case shown="\"GPU\", Default" w288 {
                      tunnel: [w290 ".raw"] -> w287
                      tunnel: w286 -> [w289 _]
                      frame "GPU", Default {
                        n67 = case shown="\"None\", Default" w289 {
                          tunnel: [".raw" "_R.raw"] -> w290
                          frame "None", Default {
                          }
                          frame "Save IQSumReal" {
                          }
                        }
                      }
                      frame "Verasonics" {
                      }
                    }
                  }
                  frame True {
                    n68 = Concatenate Strings(w301, "_I.raw") -> (w298:string)
                    n69 = Build Path(base path=w297, name or relative path=w298) -> (appended path=w296:path)
                    n70 = Open/Create/Replace File(file path (use dialog)=w296, access (0:read/write)=enum16{"read/write", "read-only", "write-only"}."read-only") -> (refnum out=w295:refnum<file>)  [unwired: 4 in, 2 out]
                  }
                }
                n71 = Concatenate Strings(w278, w273) -> (w277:string)
                n72 = Build Path(base path=w276, name or relative path=w277) -> (appended path=w283:path)
                n73 = Open/Create/Replace File(file path (use dialog)=w283, access (0:read/write)=enum16{"read/write", "read-only", "write-only"}."read-only") -> (refnum out=w282:refnum<file>, error out=w281:errorcluster)  [unwired: 4 in, 1 out]
              }
              frame "Save Img" {
                n74 = Concatenate Strings(w307, "_IMG.raw") -> (w309:string)
                n75 = Build Path(base path=w302, name or relative path=w309) -> (appended path=w306:path)
                n76 = Open/Create/Replace File(file path (use dialog)=w306, access (0:read/write)=enum16{"read/write", "read-only", "write-only"}."read-only") -> (refnum out=w305:refnum<file>, error out=w304:errorcluster)  [unwired: 4 in, 1 out]
              }
            }
            n77 = Get File Size(file=w219, error in=w218) -> (refnum out=w209:refnum<file>, size (in bytes)=w207:i64, 0:w208:errorcluster)
          }
          frame #1 {
            n78 = Index Array(array=w319) -> (element=w318:T3)  [unwired: 1 in]
            n79 = case shown="\"Save IQSum\"" w327 {
              tunnel: w328 -> [_ w343 w396 w471 w505 w588 w659 w664]
              tunnel: w318 -> [_ w355 w407 w472 w506 w589 w653 w663]
              tunnel: w315 -> [_ w341 w399 w459 w511 w586 w636 w666]
              tunnel: w313 -> [w329 w342 w400 w458 w510 w593 w635 w665]
              tunnel: w312 -> [_ w339 w398 w456 w486 w594 w652 _]
              tunnel: w326 -> [_ _ _ _ w509 w592 _ _]
              tunnel: w314 -> [_ _ _ _ w508 w591 _ _]
              tunnel: w325 -> [_ _ _ _ w507 w590 _ _]
              tunnel: w324 -> [_ _ _ _ w496 w583 _ _]
              tunnel: [_ w358 w396 w470 w499 w581 w642 w661] -> w323
              tunnel: w322 -> [_ w335 w393 w469 w493 w579 w644 _]
              tunnel: [_ w349 _ w464 w492 _ _ _] -> w321
              tunnel: [_ _ _ _ w489 w575 w638 _] -> w320
              tunnel: w317 -> [_ w334 w385 w465 w490 w574 w637 _]
              tunnel: w316 -> [_ w333 w386 _ _ _ _ _]
              tunnel: [w329 w332 w397 w455 w483 w573 w634 w660] -> w311
              tunnel: [_ w331 w394 _ _ _ _ _] -> w310
              frame "None", Default {
              }
              frame "Raw RF + time stamp" {
                w336 = i64 8 ("y")
                # "Data is transposed per frame raw"
                # "Handle 2 smps case"
                n80 = Unbundle By Name(w355) -> ("rfpts"=w356:dbl, "rflines"=w330:dbl, "Samp/Wave"=w346:dbl)
                n81 = Divide(x=w339, y=w336) -> (x/y=w340:dbl)
                n82 = Divide(x=w340, y=i64 2) -> (x/y=w337:dbl)
                n83 = Multiply(x=w356, y=w330) -> (x*y=w350:dbl)
                n84 = for {
                  N: w336 -> [_]
                  tunnel: [w362] -> w357 mode=indexing
                  shift-right: [w364] -> w332
                  shift-left: w342 -> [w361]
                  shift-right: [w365] -> _
                  shift-left: w341 -> [w360]
                  tunnel: w337 -> [w359]
                  n85 = Read from Binary File(5:i16 16 ("A/D info.# A/D bits"), 8:w361, 9:T4."little-endian" ("byte order (0:big-endian, network order)"), 10:w359, 11:w360) -> (0:w364:errorcluster, 2:w362:i16[], 3:w365:refnum<file>)  [unwired: 1 in, 1 out]
                }
                n86 = Reshape Array(w357, w335, w350) -> (w345:i16[][])
                n87 = Array Subset(array=w345, index (row)=w334, length (row)=w333) -> (w344:i16[][])  [unwired: 2 in]
                n88 = case shown="0, Default" w346 {
                  tunnel: w343 -> [w368 w376]
                  tunnel: [w367 w376] -> w358
                  tunnel: w344 -> [w370 w378]
                  tunnel: w355 -> [_ w377]
                  tunnel: [w369 w375] -> w349
                  frame 0, Default {
                    n89 = for {
                      tunnel: w370 -> [w374] mode=indexing
                      tunnel: [w373] -> w369 mode=indexing
                      tunnel: w368 -> [w372]
                      tunnel: [w371] -> w367
                      n90 = call "RF_SPW_Upsample.vi"("Header In"=w372, "RF Data In"=w374) -> ("Header Out"=w371:T1, "RF Out 2D"=w373:i16[][])  [unwired: 6 in, 2 out]
                    }
                  }
                  frame 4 {
                    n91 = for {
                      tunnel: w378 -> [w384] mode=indexing
                      tunnel: w377 -> [w383]
                      tunnel: [w379] -> w375 mode=indexing
                      n92 = Unbundle By Name(w383) -> ("rfpts"=w381:dbl, "rflines"=w380:dbl)
                      n93 = Reshape Array(w384, w381, w380) -> (w382:i16[][])
                      n94 = Transpose 2D Array(2D array=w382) -> (transposed array=w379:i16[][])
                    }
                  }
                }
                n95 = Index Array(array=w344, index (col)=w330) -> (element=w352:i16[])  [unwired: 1 in]
                n96 = Index Array(array=w344, index (col)=0 ("disabled index (row)")) -> (element=w351:i16[])  [unwired: 1 in]
                n97 = To Unsigned Word Integer(number=w351) -> (unsigned 16bit integer=w353:u16[])
                n98 = To Unsigned Word Integer(number=w352) -> (unsigned 16bit integer=w354:u16[])
                n99 = Join Numbers(hi=w353, lo=w354) -> ((hi.lo)=w347:u32[])
                n100 = Swap Words(1:w347) -> (0:w331:u32[])
              }
              frame "Time Stamps" {
                # "Data is transposed per frame raw"
                # "Handle 2 smps case"
                n101 = Unbundle By Name(w407) -> ("rfpts"=w408:dbl, "rflines"=w402:dbl)
                n102 = Multiply(x=w408, y=w402) -> (x*y=w392:dbl)
                n103 = case shown="False" FALSE {
                  tunnel: [_ w446] -> w409
                  tunnel: w400 -> [w412 w445]
                  tunnel: w399 -> [w416 w444]
                  tunnel: w398 -> [_ w443]
                  tunnel: [w415 w442] -> w397
                  tunnel: w393 -> [w417 _]
                  tunnel: w392 -> [w414 _]
                  tunnel: [w411 _] -> w390
                  tunnel: [w410 _] -> w388
                  frame False {
                    n104 = expression code="x*2"(w414) -> (w413:dbl)
                    n105 = for {
                      N: w417 -> [_]
                      tunnel: w416 -> [w428]
                      tunnel: [w423] -> w415
                      tunnel: w413 -> [w420]
                      tunnel: w412 -> [w424]
                      tunnel: [w422] -> w411 mode=indexing
                      tunnel: [w421] -> w410 mode=indexing
                      i -> [w429]
                      w418 = T4."little-endian" ("byte order (0:big-endian, network order)")
                      n106 = Multiply(x=w420, y=w429) -> (x*y=w426:dbl)
                      n107 = Set File Position(offset (in bytes) (0)=w426, refnum=w428, from (0:start)=enum16{"start", "end", "current"}."start", error in=w424) -> (refnum out=w427:refnum<file>, error out=w419:errorcluster)
                      n108 = Read from Binary File(5:i16 16 ("A/D info.# A/D bits"), 8:w419, 9:w418, 11:w427) -> (0:w435:errorcluster, 2:w422:i16, 3:w436:refnum<file>)  [unwired: 2 in, 1 out]
                      n109 = Set File Position(offset (in bytes) (0)=i64 256, refnum=w436, from (0:start)=enum16{"start", "end", "current"}."current", error in=w435) -> (refnum out=w432:refnum<file>, error out=w431:errorcluster)
                      n110 = Read from Binary File(5:i16 16 ("A/D info.# A/D bits"), 8:w431, 9:w418, 11:w432) -> (0:w423:errorcluster, 2:w421:i16)  [unwired: 2 in, 2 out]
                    }
                  }
                  frame True {
                    w438 = i64 8 ("y")
                    n111 = Divide(x=w443, y=w438) -> (x/y=w441:dbl)
                    n112 = Divide(x=w441, y=i64 2) -> (x/y=w439:dbl)
                    n113 = for {
                      N: w438 -> [_]
                      tunnel: [w447] -> w446 mode=indexing
                      shift-right: [w452] -> w442
                      shift-left: w445 -> [w450]
                      shift-right: [w453] -> _
                      shift-left: w444 -> [w449]
                      tunnel: w439 -> [w448]
                      n114 = Read from Binary File(5:i16 16 ("A/D info.# A/D bits"), 8:w450, 9:T4."little-endian" ("byte order (0:big-endian, network order)"), 10:w448, 11:w449) -> (0:w452:errorcluster, 2:w447:i16[], 3:w453:refnum<file>)  [unwired: 1 in, 1 out]
                    }
                  }
                }
                n115 = Reshape Array(w409, w393, w392) -> (w401:i16[][])
                n116 = Array Subset(array=w401, index (row)=w385, length (row)=w386) -> (w395:i16[][])  [unwired: 2 in]
                n117 = Array Subset(array=w390, index=w385) -> (w389:i16[])  [unwired: 1 in]
                n118 = Array Subset(array=w388, index=w385) -> (w387:i16[])  [unwired: 1 in]
                n119 = Index Array(array=w395, index (col)=w402) -> ()  [unwired: 1 in, 1 out]
                n120 = Index Array(array=w395, index (col)=0 ("disabled index (row)")) -> ()  [unwired: 1 in, 1 out]
                n121 = To Unsigned Word Integer(number=w389) -> (unsigned 16bit integer=w405:u16[])
                n122 = To Unsigned Word Integer(number=w387) -> (unsigned 16bit integer=w406:u16[])
                n123 = Join Numbers(hi=w405, lo=w406) -> ((hi.lo)=w403:u32[])
                n124 = Swap Words(1:w403) -> (0:w394:u32[])
              }
              frame "Save IQSumReal" {
                w460 = i64 4 ("y")
                # "Using scale values now in case GPU output is modified. Be careful of RF pts. Default IQ pt value is 1/2 of RF pts in final image.  Right now it is assumed that the Real output from GPU is sampled equal to sampling rate."
                # "Real"
                n125 = Unbundle By Name(w472) -> ("rfpts"=w468:dbl, "rflines"=w467:dbl)
                n126 = Divide(x=w456, y=w460) -> (x/y=w462:dbl)
                n127 = Divide(x=w462, y=w460) -> (x/y=w461:dbl)
                n128 = for {
                  N: w460 -> [_]
                  tunnel: [w480] -> w457 mode=indexing
                  tunnel: T4."little-endian" ("byte order (0:big-endian, network order)") -> [w478]
                  shift-right: [w482] -> _
                  shift-left: w459 -> [w477]
                  shift-right: [w481] -> w455
                  shift-left: w458 -> [w476]
                  tunnel: w461 -> [w475]
                  n129 = Read from Binary File(5:32 ("A/D info.# A/D bits"), 8:w476, 9:w478, 10:w475, 11:w477) -> (0:w481:errorcluster, 2:w480:i32[], 3:w482:refnum<file>)  [unwired: 1 in, 1 out]
                }
                n130 = Bundle By Name(cluster=w471, "A/D info.# bytes per A/D"=u16 4, "A/D info.# A/D bits"=u16 32 ("A/D info.TGC Flag")) -> (w470:T1)
                n131 = Reshape Array(w457, w469, w467, w468) -> (w466:i32[][][])
                n132 = Array Subset(array=w466, index (dim 0)=w465) -> (w464:i32[][][])  [unwired: 5 in]
              }
              frame "Save IQSum" {
                w484 = i64 4 ("y")
                # "Need to watch out for >2^31  raw file size,\nSplit raw into 4 chunks"
                # "Real"
                # "Save FIle"
                # "Pull out RcvData"
                n133 = case shown="Default" w507 {
                  tunnel: w506 -> [w527 w530]
                  tunnel: [w525 w529] -> w494
                  tunnel: w505 -> [w526 w528]
                  tunnel: [w524 w528] -> w504
                  frame "Verasonics" {
                    n134 = Unbundle By Name(w527) -> ("IQ_pts"=w525:dbl)
                    n135 = Bundle By Name(cluster=w526, "A/D info.# rf points per line"=w525) -> (w524:T1)
                  }
                  frame Default {
                    n136 = Unbundle By Name(w530) -> ("rfpts"=w529:dbl)
                  }
                }
                n137 = Divide(x=w486, y=w484) -> (x/y=w487:dbl)
                n138 = Select(t=u16 5 ("A/D info.# bytes per A/D"), s=w496, f=u16 9 ("A/D info.# bytes per A/D")) -> (s? t:f=w500:u16)
                n139 = Divide(x=w487, y=w484) -> (x/y=w485:dbl)
                n140 = case shown="False" w509 {
                  tunnel: [w539 w564] -> _
                  tunnel: [w541 w563] -> w483
                  tunnel: w511 -> [w536 w562]
                  tunnel: w510 -> [w535 w561]
                  tunnel: w508 -> [w534 _]
                  tunnel: [w540 _] -> _
                  tunnel: [w538 w553] -> w498
                  tunnel: [w537 w554] -> w497
                  tunnel: T4."little-endian" ("byte order (0:big-endian, network order)") -> [w533 w560]
                  tunnel: w485 -> [w531 w559]
                  tunnel: w484 -> [w532 w558]
                  frame True {
                    n141 = for {
                      N: w532 -> [_]
                      tunnel: [w551] -> w541
                      tunnel: [w548] -> w538 mode=concatenating
                      tunnel: [w547] -> w537 mode=concatenating
                      tunnel: w535 -> [w545]
                      shift-right: [w549] -> w539
                      shift-left: w536 -> [w546]
                      shift-right: [w550] -> w540
                      shift-left: w534 -> [w544]
                      tunnel: w533 -> [w543]
                      tunnel: w531 -> [w542]
                      w552 = 32 ("A/D info.# A/D bits")
                      n142 = Read from Binary File(5:w552, 8:w545, 9:w543, 10:w542, 11:w546) -> (2:w547:i32[], 3:w549:refnum<file>)  [unwired: 1 in, 2 out]
                      n143 = Read from Binary File(5:w552, 9:w543, 10:w542, 11:w544) -> (0:w551:errorcluster, 2:w548:i32[], 3:w550:refnum<file>)  [unwired: 2 in, 1 out]
                    }
                  }
                  frame False {
                    n144 = for {
                      N: w558 -> [_]
                      shift-right: [w572] -> w564
                      shift-left: w562 -> [w569]
                      shift-right: [w571] -> w563
                      shift-left: w561 -> [w568]
                      tunnel: w560 -> [w567]
                      tunnel: w559 -> [w566]
                      tunnel: [w565] -> w556 mode=concatenating
                      n145 = Read from Binary File(5:32 ("A/D info.# A/D bits"), 8:w568, 9:w567, 10:w566, 11:w569) -> (0:w571:errorcluster, 2:w565:i32[], 3:w572:refnum<file>)  [unwired: 1 in, 1 out]
                    }
                    n146 = Array Size(array=w556) -> (size(s)=w557:i32)
                    n147 = expression code="x/2"(w557) -> (w555:i32)
                    n148 = Split 1D Array(array=w556, index=w555) -> (first subarray=w554:i32[], second subarray=w553:i32[])
                  }
                }
                n149 = Unbundle By Name(w506) -> ("rflines"=w495:dbl)
                n150 = Bundle By Name(cluster=w504, "A/D info.# bytes per A/D"=w500, "A/D info.# A/D bits"=u16 32 ("A/D info.TGC Flag")) -> (w499:T1)
                n151 = case shown="False" w496 {
                  tunnel: w498 -> [w518 _]
                  tunnel: w497 -> [w517 w523]
                  tunnel: w495 -> [w513 w522]
                  tunnel: w494 -> [w512 w521]
                  tunnel: w493 -> [w515 w519]
                  tunnel: [w514 _] -> w491
                  tunnel: [_ w520] -> w492
                  frame False {
                    n152 = Re/Im To Complex(1:w518, 2:w517) -> (0:w516:cdb[])
                    n153 = Reshape Array(w516, w515, w513, w512) -> (w514:cdb[][][])
                  }
                  frame True {
                    n154 = Reshape Array(w523, w519, w522, w521) -> (w520:i32[][][])
                  }
                }
                n155 = Array Subset(array=w491, index (dim 0)=w490) -> (w489:cdb[][][])  [unwired: 5 in]
              }
              frame "Save IQAll" {
                # "Using scale values now in case GPU output is modified."
                # "Real"
                # "Save FIle"
                n156 = case shown="False" w592 {
                  tunnel: [w609 w623] -> _
                  tunnel: [w616 w622] -> w573
                  tunnel: w594 -> [_ w632]
                  tunnel: w586 -> [w615 w621]
                  tunnel: w593 -> [w614 w620]
                  tunnel: w591 -> [w608 _]
                  tunnel: [w610 _] -> _
                  tunnel: [w605 w626] -> w580
                  frame True {
                    w603 = T4."little-endian" ("byte order (0:big-endian, network order)")
                    w604 = -1
                    w617 = 32 ("A/D info.# A/D bits")
                    w611 = enum16{"start", "end", "current"}."start" ("from (0:start)")
                    n157 = Set File Position(refnum=w615, from (0:start)=w611, error in=w614) -> (refnum out=w612:refnum<file>, error out=w613:errorcluster)  [unwired: 1 in]
                    n158 = Read from Binary File(5:w617, 8:w613, 9:w603, 10:w604, 11:w612) -> (2:w607:i32[], 3:w609:refnum<file>)  [unwired: 1 in, 2 out]
                    n159 = Set File Position(refnum=w608, from (0:start)=w611) -> (refnum out=w618:refnum<file>, error out=w619:errorcluster)  [unwired: 2 in]
                    n160 = Read from Binary File(5:w617, 8:w619, 9:w603, 10:w604, 11:w618) -> (0:w616:errorcluster, 2:w606:i32[], 3:w610:refnum<file>)  [unwired: 1 in, 1 out]
                    n161 = Re/Im To Complex(1:w606, 2:w607) -> (0:w605:cdb[])
                  }
                  frame False {
                    n162 = Divide(x=w632, y=i64 8) -> (x/y=w629:dbl)
                    n163 = Read from Binary File(5:32 ("A/D info.# A/D bits"), 8:w620, 9:T4."little-endian" ("byte order (0:big-endian, network order)"), 10:-1, 11:w621) -> (0:w622:errorcluster, 2:w630:i32[], 3:w623:refnum<file>)  [unwired: 1 in, 1 out]
                    n164 = Split 1D Array(array=w630, index=w629) -> (first subarray=w628:i32[], second subarray=w627:i32[])
                    n165 = Re/Im To Complex(1:w627, 2:w628) -> (0:w626:cdb[])
                  }
                }
                n166 = case shown="Default" w590 {
                  tunnel: w589 -> [w599 w602]
                  tunnel: [w597 w601] -> w577
                  tunnel: w588 -> [w598 w600]
                  tunnel: [w596 w600] -> w587
                  frame "Verasonics" {
                    n167 = Unbundle By Name(w599) -> ("IQ_pts"=w597:dbl)
                    n168 = Bundle By Name(cluster=w598, "A/D info.# rf points per line"=w597) -> (w596:T1)
                  }
                  frame Default {
                    n169 = Unbundle By Name(w602) -> ("rfpts"=w601:dbl)
                  }
                }
                n170 = Select(t=u16 4 ("A/D info.# bytes per A/D"), s=w583, f=u16 9 ("A/D info.# bytes per A/D")) -> (s? t:f=w582:u16)
                n171 = Bundle By Name(cluster=w587, "A/D info.# bytes per A/D"=w582, "A/D info.# A/D bits"=u16 32 ("A/D info.TGC Flag")) -> (w581:T1)
                n172 = Unbundle By Name(w589) -> ("rflines"=w578:dbl)
                n173 = Reshape Array(w580, w579, w578, w577) -> (w576:cdb[][][])
                n174 = Array Subset(array=w576, index (dim 0)=w574) -> (w575:cdb[][][])  [unwired: 5 in]
              }
              frame "unused" {
                w654 = 2.0  # double
                n175 = Unbundle By Name(w653) -> ("IQ_pts"=w640:dbl, "rflines"=w641:dbl)
                n176 = Divide(x=w652, y=i64 8) -> (x/y=w647:dbl)
                n177 = Multiply(x=w654, y=w640) -> (x*y=w655:dbl)
                n178 = Read from Binary File(5:32 ("A/D info.# A/D bits"), 8:w635, 9:T4."little-endian" ("byte order (0:big-endian, network order)"), 10:-1 ("count (1)"), 11:w636) -> (0:w634:errorcluster, 2:w648:i32[])  [unwired: 1 in, 2 out]
                n179 = Bundle By Name(cluster=w659, "A/D info.# rf points per line"=w655, "A/D info.# bytes per A/D"=u16 9, "A/D info.# A/D bits"=u16 32 ("A/D info.TGC Flag")) -> (w642:T1)
                n180 = Split 1D Array(array=w648, index=w647) -> (first subarray=w650:i32[], second subarray=w649:i32[])
                n181 = Re/Im To Complex(1:w649, 2:w650) -> (0:w643:cdb[])
                n182 = Reshape Array(w643, w644, w641, w640) -> (w639:cdb[][][])
                n183 = Array Subset(array=w639, index (dim 0)=w637) -> (w638:cdb[][][])  [unwired: 5 in]
              }
              frame "Save Img" {
                n184 = Unbundle By Name(w663) -> ("IQPage"=w662:dbl)
                n185 = case shown="1" w662 {
                  tunnel: w663 -> [_ w680]
                  tunnel: w666 -> [w668 w678]
                  tunnel: w665 -> [w667 w677]
                  tunnel: [w668 w676] -> _
                  tunnel: [w667 w669] -> _
                  tunnel: w664 -> [_ w674]
                  tunnel: [_ w670] -> w661
                  tunnel: [w667 w669] -> w660
                  frame 0, Default {
                  }
                  frame 1 {
                    # "Only save page 1 cases. This is nod to Doppler"
                    # "Save FIle"
                    # "Pull out RcvData"
                    n186 = Unbundle By Name(w680) -> ("IQ_pts"=w673:dbl, "rflines"=w679:dbl)
                    n187 = Set File Position(refnum=w678, from (0:start)=enum16{"start", "end", "current"}."current", error in=w677) -> (refnum out=w681:refnum<file>, error out=w682:errorcluster)  [unwired: 1 in]
                    n188 = Bundle By Name(cluster=w674, "A/D info.# rf points per line"=w673, "A/D info.# bytes per A/D"=u16 4, "A/D info.# A/D bits"=i16 32) -> (w670:T1)
                    n189 = Multiply(x=w673, y=w679) -> (x*y=w683:dbl)
                    n190 = Read from Binary File(5:32 ("A/D info.# A/D bits"), 8:w682, 10:w683, 11:w681) -> (0:w669:errorcluster, 3:w676:refnum<file>)  [unwired: 2 in, 2 out]
                  }
                }
              }
            }
          }
          frame #2 {
            n191 = case shown="\"Raw RF + time stamp\", Default" w689 {
              tunnel: w685 -> [_ w693]
              tunnel: w686 -> [_ w692]
              tunnel: w688 -> [_ w691]
              tunnel: w687 -> [_ w690]
              frame "None" {
              }
              frame "Raw RF + time stamp", Default {
                n192 = case shown="True" w691 {
                  tunnel: w690 -> [_ w694]
                  frame False {
                  }
                  frame True {
                    n193 = Close File(refnum=w694) -> ()  [unwired: 1 in, 2 out]
                  }
                }
                n194 = Close File(refnum=w692, error in=w693) -> ()  [unwired: 2 out]
              }
            }
          }
        }
      }
    }
  }
  "Header Out" <- w38
  "RcvBuff 3" <- w19
  "output array" <- w20
  n195 = Index Array(array=w3) -> (element=w5:u32)  [unwired: 1 in]
  n196 = Subtract(x=w3, y=w5) -> (x-y=w6:u32[])
  n197 = Divide(x=w6, y=sgl 40.0) -> (x/y=w2:sgl[])
  "time stamp" <- w2
  n198 = Index Array(array=w19) -> (element=w18:cdb[][])  [unwired: 3 in]
  n199 = Absolute Value(x=w18) -> (abs(x)=w17:dbl[][])
  n200 = Array Size(array=w2) -> (size(s)=w8:i32)
  n201 = expression code="20*log(abs(X))"(w17) -> (→"Raw data":dbl[][])
  n202 = Decrement(x=w8) -> (x-1=w7:i32)
  n203 = for {
    N: w7 -> [_]
    tunnel: w2 -> [w697] mode=indexing
    tunnel: w2 -> [w699]
    tunnel: [w696] -> w1 mode=indexing
    i -> [w695]
    n204 = Increment(x=w695) -> (x+1=w700:i32)
    n205 = Index Array(array=w699, index=w700) -> (element=w698:sgl)
    n206 = Subtract(x=w698, y=w697) -> (x-y=w696:sgl)
  }
  "time diff (25 us time steps)" <- w1
